vi "Obtain Station Model.vi"(0 "Session Handle in":T2, 11 "error in (no error)":errorcluster) -> (4 "Session Handle out":T2, 6 "Station Model":T1, 15 "error out":errorcluster)   [LabVIEW 2020, in "TSS.lvlib" / "Engine.lvclass"]
uses:
  Engine.lvclass
  Typedefs/Session Handle.ctl
  SequenceFile/Typedefs/Session Handle.ctl
  SequenceFile/SequenceFile.lvclass
  Engine.lvclass/Engine.ctl
  Data Types/File Load Options.ctl
  TSS.lvlib
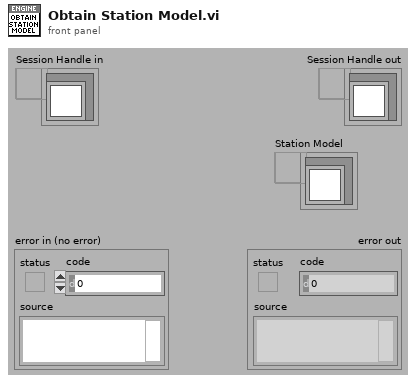
[diagram p1: front panel]
types:
  T1 = typedef "TSS.lvlib/SequenceFile.lvclass/Session Handle.ctl" = refnum<data-value>
  T2 = typedef "TSS.lvlib/Engine.lvclass/Session Handle.ctl" = refnum<data-value>
  T3 = typedef "TSS.lvlib/File Load Options.ctl" = cluster{"Use Search Dirs? (T)":bool, "Conflict as Error? (T)":bool, "Check Station Model? (F)":bool, "Preload Modules? (T)":bool, "Skip Load Callback? (F)":bool, "Reload if Loaded? (F)":bool}
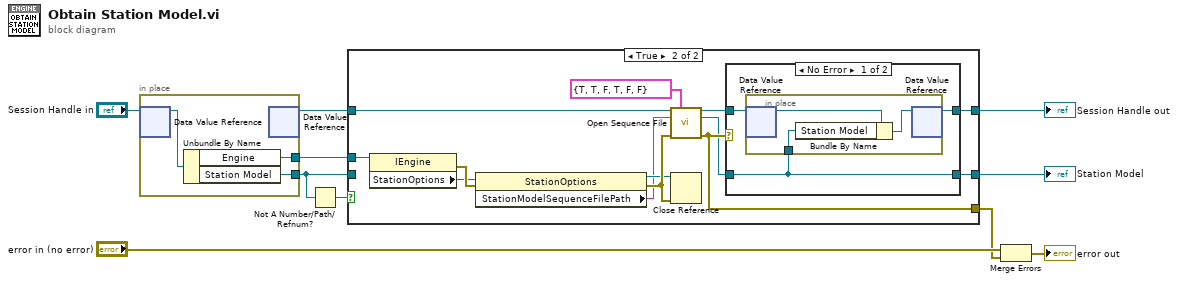
[diagram p0: block diagram]
diagram:
  n1 = in-place {
    in-place-border: [w12] -> w6
    in-place-border: [w11] -> w5
    n2 = in-place-dvr #1("Session Handle in") -> (w13:refnum<class "Engine.lvclass">)  [unwired: 1 out]
    n3 = Unbundle By Name(w13) -> ("Engine"=w11:refnum<k7>, "Station Model"=w12:T1)
    n4 = in-place-dvr #1() -> (w8:T2)  [unwired: 1 in, 1 out]
  }
  n5 = Not A Number/Path/Refnum?(number/path/refnum=w6) -> (NaN/Path/Refnum?=w7:bool)
  n6 = case shown="True" w7 {
    tunnel: w8 -> [w14 w23]
    tunnel: w6 -> [w15 _]
    tunnel: w5 -> [_ w24]
    tunnel: [w15 w19] -> w4
    tunnel: [w14 w18] -> w3
    tunnel: [_ w17] -> w1
    frame False {
    }
    frame True {
      n7 = property class="IEngine"(reference=w24) -> (error out=w27:errorcluster, "StationOptions"=w26:refnum<k7>)  [unwired: 1 in, 1 out]
      n8 = property class="StationOptions"(reference=w26, error in=w27) -> (reference out=w25:refnum<k7>, error out=w28:errorcluster, "StationModelSequenceFilePath"=w21:string)
      n9 = call "Open Sequence File.vi"("Session Handle in"=w23, "Load Options"=T3 {"Use Search Dirs? (T)"=TRUE, "Conflict as Error? (T)"=TRUE, "Check Station Model? (F)"=FALSE, "Preload Modules? (T)"=TRUE, "Skip Load Callback? (F)"=FALSE, "Reload if Loaded? (F)"=FALSE}, "File Path"=w21, "error in (no error)"=w28) -> ("Session Handle out"=w20:T2, "SequenceFile"=w16:T1, "error out"=w17:errorcluster)  [unwired: 9 in]
      n10 = Close Reference(reference=w25, error in (no error)=w28) -> ()  [unwired: 1 out]
      n11 = case shown="No Error" w17 {
        tunnel: w20 -> [w31 w35]
        tunnel: w16 -> [w30 _]
        tunnel: [w30 _] -> w19
        tunnel: [w29 w35] -> w18
        frame No Error {
          n12 = in-place {
            in-place-border: w30 -> [w33]
            n13 = in-place-dvr #2(w31) -> (w34:refnum<class "Engine.lvclass">)  [unwired: 1 out]
            n14 = Bundle By Name(cluster=w34, "Station Model"=w33) -> (w32:refnum<class "Engine.lvclass">)
            n15 = in-place-dvr #2(w32) -> (w29:T2)  [unwired: 1 out]
          }
        }
        frame Error {
        }
      }
    }
  }
  "Session Handle out" <- w3
  "Station Model" <- w4
  n16 = Merge Errors("error in (no error)", w1) -> (→"error out":errorcluster)
